vi "LVClass_HasoField ctor.vi"(0 "HasoField (const)":refnum<class "HasoField.lvclass">, 1 "wavelenght nm":dbl, 2 "haso_config_file_path":path, 5 "HasoSlopes":refnum<class "HasoSlopes.lvclass">, 7 "Phase":refnum<class "Phase.lvclass">, 9 "radius_of_curvature _ mm":dbl, 11 "error in (no error)":errorcluster, 12 "oversampling_level":u8) -> (3 "wavelenght out":dbl, 4 "HasoField (new)":refnum<class "HasoField.lvclass">, 6 "HasoSlopes (dup)":refnum<class "HasoSlopes.lvclass">, 8 "Phase (dup)":refnum<class "Phase.lvclass">, 15 "error out":errorcluster)   [LabVIEW 2020, in "HasoField.lvclass"]
doc: "HasoField constructor from HasoSlopes and phase.\n\n--------------------------------------------------------------------------------\n\n<B>HasoFieldIn </B> : Constant Pointer to HasoField object.\n<B>HasoFieldOut </B> : Constant Pointer to HasoField object.\n<B>haso_config_file_path </B> : Absolute path to Haso configuration file.\n<B>HasoSlopes </B> : HasoSlopes object.\n<B>Phase </B> : phase object.\n<B>radius_of_curvature </B> : Radius of curvature (mm).\n<B>wavelength </B> : Wavelenght of the source used to compute the HasoSlopes (nm).\n<B>oversampling_level </B> : Increment of oversampling level.\n<B>ErrorIn </B> : Error\n<B>ErrorOut </B> : Error\n\n--------------------------------------------------------------------------------"
uses:
  HasoField.lvclass
  HasoSlopes/HasoSlopes.lvclass
  Phase/Phase.lvclass
  Controls/Handle creation.ctl
  HasoField.lvclass/HasoField.ctl
  Phase/LVClasse_Phase Read SurfaceFloatWithPupil.vi
  HasoSlopes/LVClass_HasoSlopes Read HasoSlopes _ property.vi
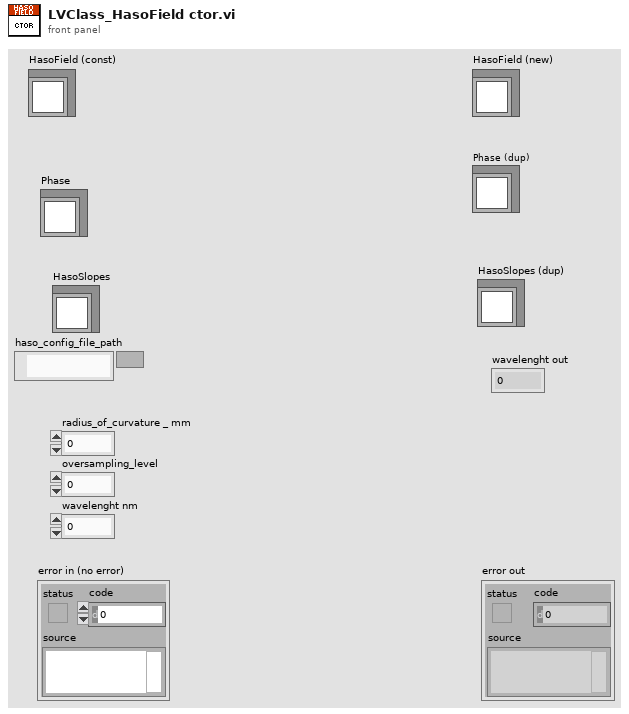
[diagram p1: front panel]
types:
  T1 = typedef "Handle creation.ctl" = enum16{"By ctor", "By write function"}
  T2 = typedef "ClassID.ctl" = i64
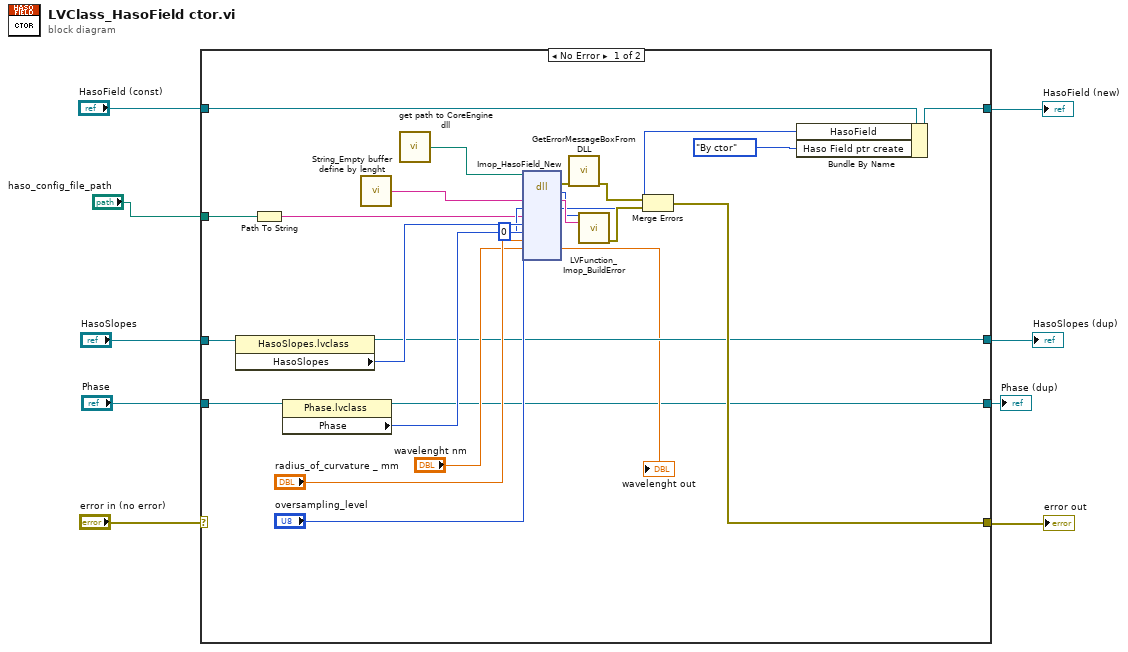
[diagram p0: block diagram]
diagram:
  n1 = case shown="No Error" "error in (no error)" {
    selector: "error in (no error)" -> [_ w38]
    tunnel: [w25 w38] -> w8
    tunnel: [w18 w37] -> w6
    tunnel: "HasoField (const)" -> [w19 w37]
    tunnel: "HasoSlopes" -> [w27 w36]
    tunnel: "Phase" -> [w26 w35]
    tunnel: [w14 w36] -> w4
    tunnel: "haso_config_file_path" -> [w11 _]
    tunnel: [w10 w35] -> w1
    frame No Error {
      n2 = property class="HasoSlopes.lvclass"(reference=w27) -> (reference out=w14:refnum<class "HasoSlopes.lvclass">, "HasoSlopes"=w24:T2)  [unwired: 1 in, 1 out]
      n3 = Path To String(path=w11) -> (string=w12:string)
      n4 = property class="Phase.lvclass"(reference=w26) -> (reference out=w10:refnum<class "Phase.lvclass">, "Phase"=w23:T2)  [unwired: 1 in, 1 out]
      n5 = call "String_Empty buffer define by lenght.vi"() -> ("Empty buffer"=w34:string)  [unwired: 1 in]
      n6 = call "get path to CoreEngine dll.vi"() -> ("path to wavekit library"=w31:path)  [unwired: 14 in, 1 out]
      n7 = dll-call lib="D:/soft/HASO_v3/SVN_trunk/ImOpCoreEngine4_LV2011/DLLs/c_interface_vc100.dll" fn="Imop_HasoField_New"(path in=w31, "message"=w34, "hasofield"=0, "haso_config_file_path"=w12, "HasoSlopes"=w24, "Phase"=w23, "radius_of_curvature"="radius_of_curvature _ mm", "wavelenght"="wavelenght nm", "oversampling_level"="oversampling_level") -> (error out=w30:errorcluster, "return type"=w32:i32, "message"=w33:string, "hasofield"=w17:i64, "wavelenght"=→"wavelenght out":dbl)  [unwired: 7 in, 1 out]
      n8 = call "GetErrorMessageBoxFromDLL.vi"("error IN"=w30) -> ("error OUT"=w29:errorcluster)  [unwired: 10 in]
      n9 = call "LVFunction_Imop_BuildError.vi"("code"=w32, "String to Prepend to source (\"\")"=w33) -> ("error out"=w28:errorcluster)  [unwired: 13 in]
      n10 = Merge Errors(w29, w28) -> (w25:errorcluster)
      n11 = Bundle By Name(cluster=w19, "HasoField"=w17, "Haso Field ptr create"=Handle_creation."By ctor") -> (w18:refnum<class "HasoField.lvclass">)
    }
    frame Error {
    }
  }
  "error out" <- w8
  "HasoField (new)" <- w6
  "HasoSlopes (dup)" <- w4
  "Phase (dup)" <- w1
